vi "test_AK TCP Read.vi"(8 "error in (no error)":errorcluster, 11 "TestCase in":refnum<class "Ethernet Protocol Tests.lvclass">) -> (0 "error out":errorcluster, 3 "TestCase out":refnum<class "Ethernet Protocol Tests.lvclass">)   [LabVIEW 2019, in "Ethernet Protocol Tests.lvclass"]
uses:
  Ethernet Protocol Tests.lvclass
  Listener/Listener.lvclass
  Listener/ListenerClassControls/Operation.ctl
  AK TCP/AK TCP.lvclass
  D:/GitRepository/niveristand-instrument-addon-classes/Source/Protocols/TCP/TCP.lvclass
  D:/GitRepository/niveristand-instrument-addon-classes/Source/Protocols/Protocol Parent/Protocol Parent.lvclass
  Protocol Parent/Methods/Read Parameter.ctl
  TCP/TCP.lvclass/TCP.ctl
  AK TCP/AK TCP.lvclass/AK TCP.ctl
  Constants.vi
  <vilib>/addons/_JKI Toolkits/VI Tester/TestCase.llb/TestCase.lvclass
  TCP/TCP.lvclass
  Protocol Parent/Protocol Parent.lvclass
  C:/Program Files (x86)/National Instruments/LabVIEW 2019/vi.lib/addons/_JKI Toolkits/VI Tester/TestCase.llb/TestCase.lvclass
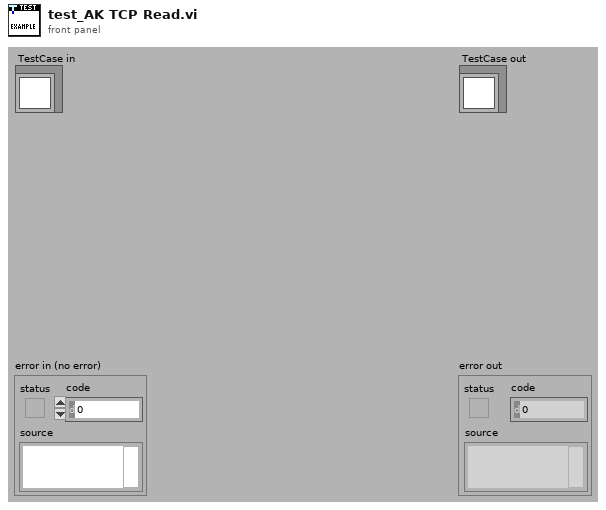
[diagram p1: front panel]
types:
  T1 = typedef "Protocols.lvlib/Protocol Parent.lvclass/Read Parameter.ctl" = cluster{"Wait Type":enum16{"Byte Count", "Wait sec"}, "Wait Value":dbl}
  T2 = typedef "Listener.lvclass/Operation.ctl" = enum16{"Read", "Write"}
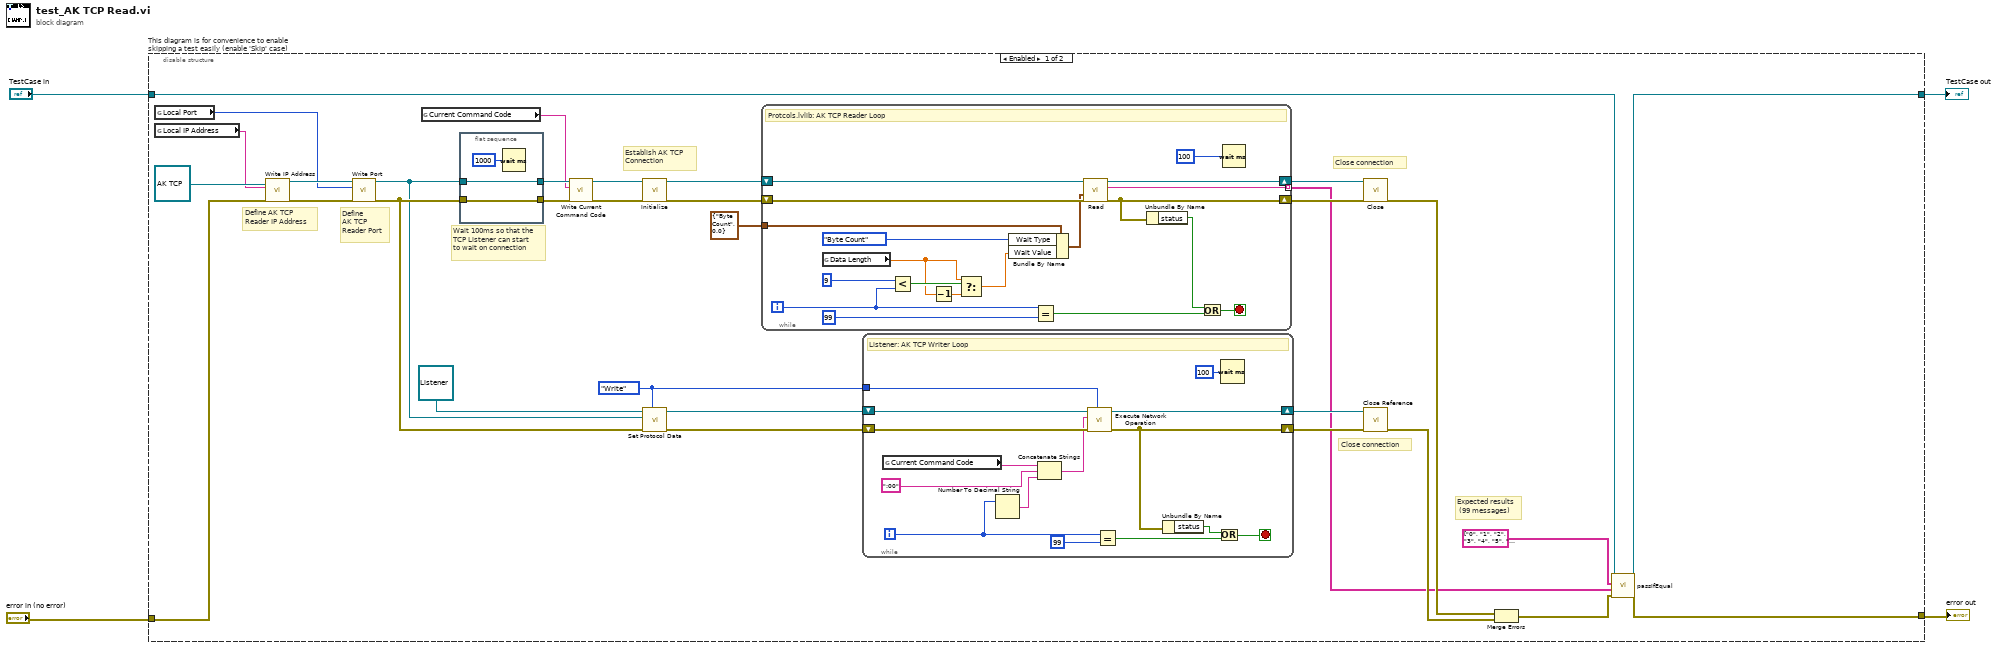
[diagram p0: block diagram]
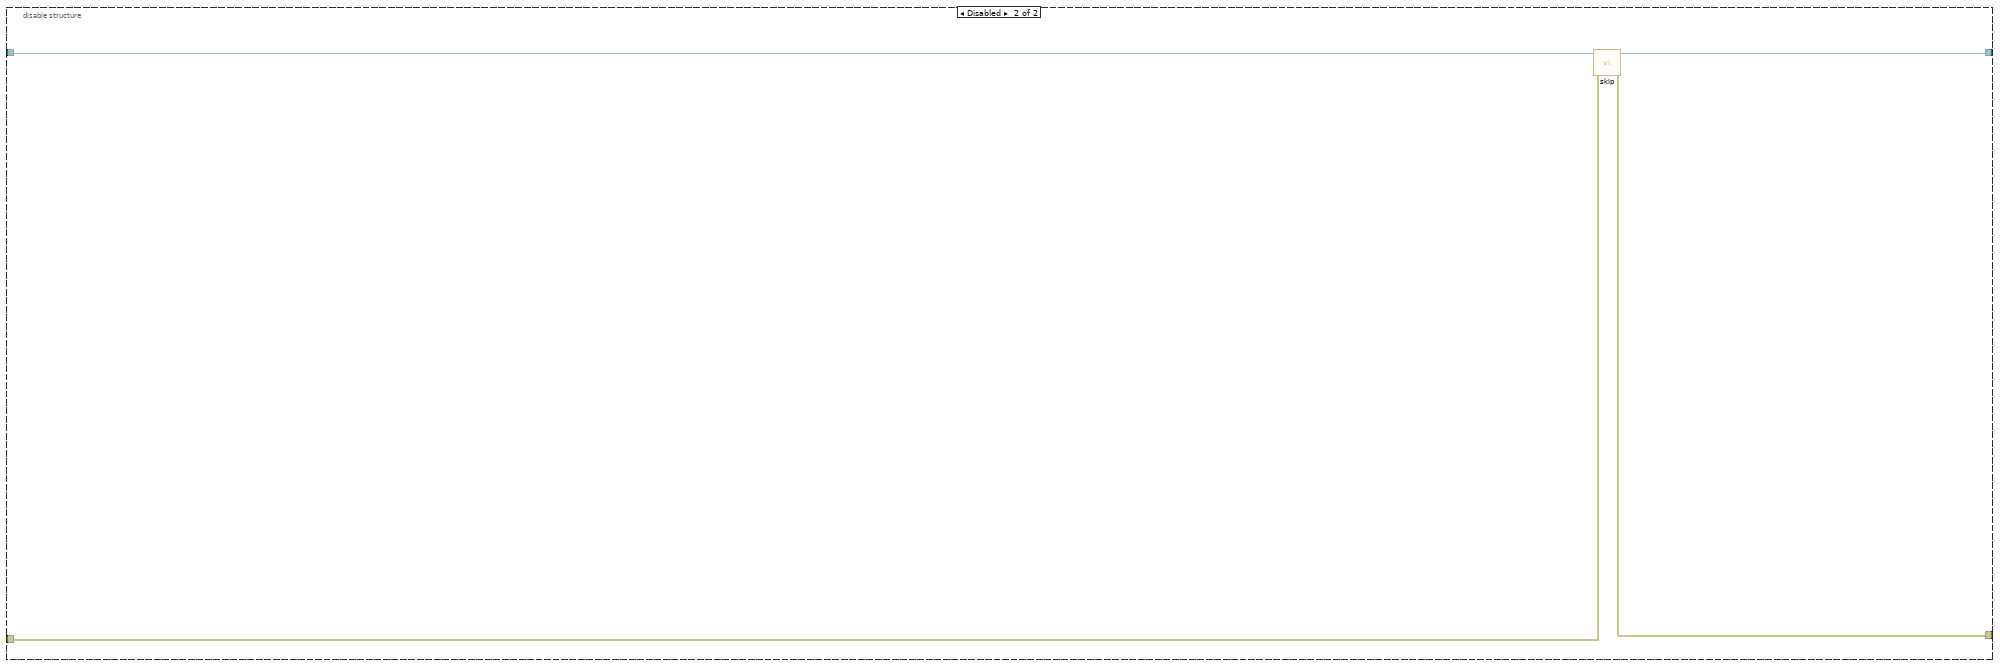
[diagram p2: hidden frame]
diagram:
  n1 = disable-structure "This diagram is for convenience to enable skipping a test easily (enable 'Skip' case)" shown="Enabled" {
    disable-tunnel: "TestCase in" -> [w36 w77]
    disable-tunnel: [w35 w75] -> w1
    disable-tunnel: [w34 w76] -> w3
    disable-tunnel: "error in (no error)" -> [w31 w74]
    frame Enabled {
      w26 = Operation."Write" ("Operation")
      # "Wait 100ms so that the\nTCP Listener can start \nto wait on connection"
      # "Establish AK TCP \nConnection"
      # "Close connection"
      # "Close connection"
      # "Expected results\n (99 messages)"
      # "Define \nAK TCP \nReader Port"
      # "Define AK TCP \nReader IP Address"
      n2 = global read "Constants.vi" "Local Port"() -> (w6:u16)
      n3 = global read "Constants.vi" "Local IP Address"() -> (w7:string)
      n4 = call "Write IP Address.vi"("error in (no error)"=w31, "IP Address"=w7, "Ethernet in"=refnum<class "AK TCP.lvclass"> refnum ("Protocols.lvlib:AK TCP.lvclass")) -> ("error out"=w32:errorcluster, "Ethernet out"=w33:refnum<class "AK TCP.lvclass">)  [unwired: 7 in]
      n5 = call "Write Port.vi"("error in (no error)"=w32, "Port"=w6, "Ethernet in"=w33) -> ("error out"=w12:errorcluster, "Ethernet out"=w10:refnum<class "AK TCP.lvclass">)  [unwired: 7 in]
      n6 = global read "Constants.vi" "Current Command Code"() -> (w5:string)
      n7 = flat-sequence {
        tunnel: w12 -> [w39]
        tunnel: [w39] -> w11
        tunnel: w10 -> [w38]
        tunnel: [w38] -> w9
        frame #0 {
          n8 = Wait (ms)(milliseconds to wait=u32 1000) -> ()  [unwired: 1 out]
        }
      }
      n9 = call "Write Current Command Code.vi"("error in (no error)"=w11, "Current Command Code"=w5, "AK TCP in"=w9) -> ("error out"=w16:errorcluster, "AK TCP out"=w15:refnum<class "AK TCP.lvclass">)  [unwired: 7 in]
      n10 = call-dynamic "Initialize.vi"("error in (no error)"=w16, "Ethernet in"=w15) -> ("error out"=w14:errorcluster, "Ethernet out"=w13:refnum<class "AK TCP.lvclass">)  [unwired: 8 in]
      n11 = call "Set Protocol Data.vi"("Operation"=w26, "error in (no error)"=w12, "Protocols.lvlib:Protocol Parent.lvclass"=w10, "Listener In.lvclass"=refnum<class "Listener.lvclass"> refnum ("Listener.lvclass")) -> ("error out"=w27:errorcluster, "Listener Out.lvclass"=w28:refnum<class "Listener.lvclass">)  [unwired: 6 in]
      n12 = while {
        shift-right: [w66] -> w22
        shift-left: w14 -> [w67]
        shift-right: [w65] -> w21
        shift-left: w13 -> [w68]
        tunnel: [w64] -> w17 mode=indexing
        tunnel: T1 {"Wait Type"=enum."Byte Count", "Wait Value"=0.0} ("Read Parameter") -> [w57]
        i -> [w61]
        stop <- w72 stop-if-true
        # "Protcols.lvlib: AK TCP Reader Loop"
        n13 = global read "Constants.vi" "Data Length"() -> (w55:dbl)
        n14 = Less?(x=9, y=w61) -> (x < y?=w59:bool)
        n15 = Decrement(x=w55) -> (x-1=w56:dbl)
        n16 = Select(t=w55, s=w59, f=w56) -> (s? t:f=w58:dbl)
        n17 = Bundle By Name(cluster=w57, "Wait Type"=enum16{"Byte Count", "Wait sec"}."Byte Count", "Wait Value"=w58) -> (w62:T1)
        n18 = Equal?(x=w61, y=99 ("x")) -> (x = y?=w73:bool)
        n19 = call-dynamic "Read.vi"("error in (no error)"=w67, "Variant"=w62, "AK TCP in"=w68) -> ("error out"=w66:errorcluster, "String"=w64:string, "AK TCP out"=w65:refnum<class "AK TCP.lvclass">)  [unwired: 6 in]
        n20 = Unbundle By Name(w66) -> ("status"=w69:bool)
        n21 = Or(x=w69, y=w73) -> (x .or. y?=w72:bool)
        n22 = Wait (ms)(milliseconds to wait=u32 100) -> ()  [unwired: 1 out]
      }
      n23 = while {
        shift-right: [w46] -> w24
        shift-left: w27 -> [w54]
        shift-right: [w45] -> w25
        shift-left: w28 -> [w53]
        tunnel: w26 -> [w48]
        i -> [w43]
        stop <- w51 stop-if-true
        # "Listener: AK TCP Writer Loop"
        n24 = global read "Constants.vi" "Current Command Code"() -> (w40:string)
        n25 = Number To Decimal String(number=w43) -> (decimal integer string=w42:string)  [unwired: 1 in]
        n26 = Concatenate Strings(w40, ":00", w42) -> (w41:string)
        n27 = call "Execute Network Operation.vi"("Operation"=w48, "error in (no error)"=w54, "Message"=w41, "Listener In.lvclass"=w53) -> ("error out"=w46:errorcluster, "Listener Out.lvclass"=w45:refnum<class "Listener.lvclass">)  [unwired: 6 in]
        n28 = Equal?(x=w43, y=99 ("x")) -> (x = y?=w50:bool)
        n29 = Unbundle By Name(w46) -> ("status"=w52:bool)
        n30 = Or(x=w52, y=w50) -> (x .or. y?=w51:bool)
        n31 = Wait (ms)(milliseconds to wait=u32 100) -> ()  [unwired: 1 out]
      }
      n32 = call-dynamic "Close.vi"("error in (no error)"=w22, "Ethernet in"=w21) -> ("error out"=w20:errorcluster)  [unwired: 8 in, 1 out]
      n33 = call "Close Reference.vi"("error in (no error)"=w24, "Listener In.lvclass"=w25) -> ("error out"=w23:errorcluster)  [unwired: 9 in]
      n34 = Merge Errors(w20, w23) -> (w30:errorcluster)
      n35 = call-dynamic "passIfEqual.vi"("error in (no error)"=w30, "y"=w17, "x"=string[] ["0", "1", "2", "3", "4", "5", "6", "7", "8", "9", "10", "11", "12", "13", "14", "15", "16", "17", "18", "19", "20", "21", "22", "23", "24", "25", "26", "27", "28", "29", "30", "31", "32", "33", "34", "35", "36", "37", "38", "39", "40", "41", "42", "43", "44", "45", "46", "47", "48", "49", "50", "51", "52", "53", "54", "55", "56", "57", "58", "59", "60", "61", "62", "63", "64", "65", "66", "67", "68", "69", "70", "71", "72", "73", "74", "75", "76", "77", "78", "79", "80", "81", "82", "83", "84", "85", "86", "87", "88", "89", "90", "91", "92", "93", "94", "95", "96", "97", "98", "99"] ("Array"), "TestCase in"=w36) -> ("error out"=w34:errorcluster, "TestCase out"=w35:refnum<class "Ethernet Protocol Tests.lvclass">)  [unwired: 6 in]
    }
    frame Disabled {
      # "skip test result while test is under development"
      n36 = call <vilib>:"skip.vi"("error in (no error)"=w74, "TestCase in"=w77) -> ("error out"=w76:errorcluster, "TestCase out"=w75:refnum<class "Ethernet Protocol Tests.lvclass">)  [unwired: 8 in]
    }
  }
  "error out" <- w3
  "TestCase out" <- w1
